vi "isItemActive.vi"(8 "error in (no error)":errorcluster, 10 "rowIndex":i32, 11 "ScriptEditorV2 in":refnum<class "ScriptEditorV2.lvclass">) -> (0 "error out":errorcluster, 2 "active":bool, 3 "ScriptEditorV2 out":refnum<class "ScriptEditorV2.lvclass">)   [LabVIEW 2009, in "Views.lvlib" / "ScriptEditor.lvlib" / "ScriptEditorV2.lvclass"]
uses:
  ScriptEditorV2.lvclass
  ScriptEditorV2.lvclass/ScriptEditorV2.ctl
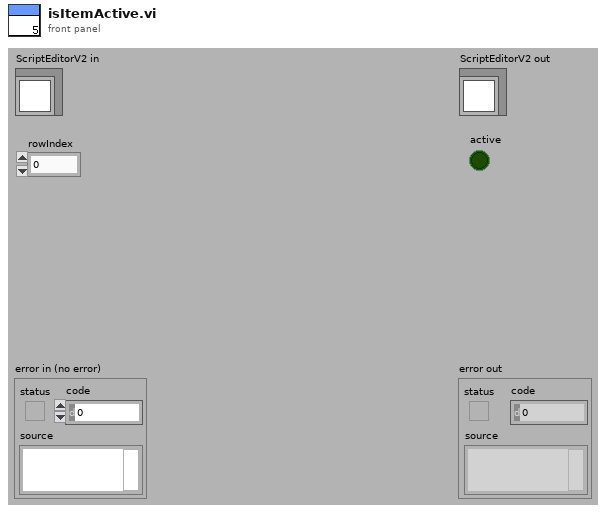
[diagram p1: front panel]
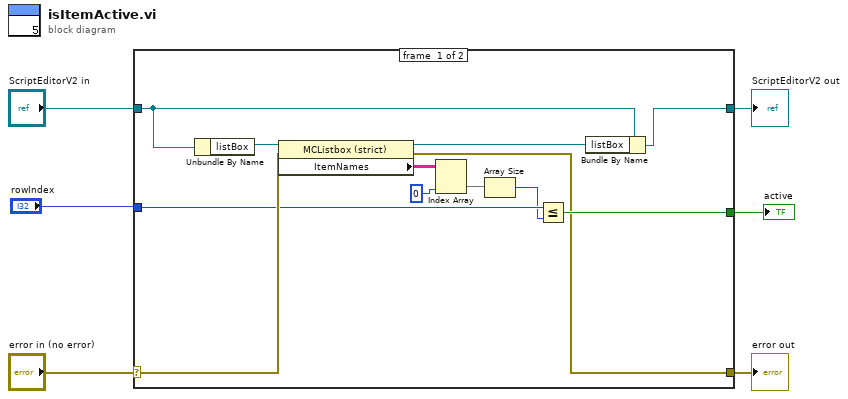
[diagram p0: block diagram]
diagram:
  n1 = case shown="No Error" "error in (no error)" {
    selector: "error in (no error)" -> [w17 w20]
    tunnel: [w10 w20] -> w5
    tunnel: [w7 w19] -> w3
    tunnel: "ScriptEditorV2 in" -> [w8 w19]
    tunnel: "rowIndex" -> [w13 _]
    tunnel: [w11 _] -> w1
    frame #0 {
      n2 = Unbundle By Name(w8) -> ("listBox"=w18:refnum<vi>)
      n3 = property class="MCListbox (strict)"(reference=w18, error in=w17) -> (reference out=w9:refnum<vi>, error out=w10:errorcluster, "ItemNames"=w16:string[][])
      n4 = Index Array(array=w16, index (col)=0) -> (element=w14:string[])  [unwired: 1 in]
      n5 = Array Size(array=w14) -> (size(s)=w12:i32)
      n6 = Less Or Equal?(x=w13, y=w12) -> (x <= y?=w11:bool)
      n7 = Bundle By Name(cluster=w8, "listBox"=w9) -> (w7:refnum<class "ScriptEditorV2.lvclass">)
    }
    frame #1 {
    }
  }
  "error out" <- w5
  "ScriptEditorV2 out" <- w3
  "active" <- w1
